vi "Read from memory.vi"(8 "input valid":bool=TRUE, 10 "Address":u32, 11 "Memory item":refnum<k21>="PID Output I") -> (0 "output valid":bool=TRUE, 2 "Address out":u32, 3 "Value out":fxp<+/-,32,14>)   [LabVIEW 2018]
uses:
  <vilib>/rvi/DataTransferAndStorage/Container/Common/niFpgaContainerExecOnDevCompGetState.vi
  <vilib>/rvi/Emulation/niFpgaEmulationIsFPGAContextNoSignature.vi
  <vilib>/rvi/DataTransferAndStorage/Container/Common/niFpgaContainerGetUniqueNameForEmu.vi
  <vilib>/rvi/Emulation/niFpgaProcessEmulError.vi
  <vilib>/rvi/Emulation/niFpgaSctlEmulationGetInTimedLoop.vi
  <vilib>/rvi/errors/nirviReportUnexpectedCaseInternalError (U32).vi
  <vilib>/rvi/Memory/Memory_Emulation/niFpgaMemoryEmulationCacheClearOnFirstRun.vi
  <vilib>/rvi/Memory/Memory_Emulation/nirvimemoryEmulationManagerCache_MakeExclusive.vi
  <vilib>/rvi/Memory/Memory_Emulation/niFpgaMemoryEmulationValidateCache.vi
  <vilib>/rvi/Memory/Memory_Emulation/nirvimemoryEmulationManagerCache_InsertValue.vi
  <vilib>/Utility/error.llb/Clear Errors.vi
  <vilib>/rvi/Memory/Memory_Emulation/nirvimemoryEmulationManagerCache_ReleaseExclusive.vi
  <vilib>/rvi/Memory/Memory_Emulation/nirvimemoryEmulationManagerCache_GetValue.vi
  <vilib>/rvi/Memory/Memory_Emulation/nirvimemoryEmulationManagerCache_SetValue.vi
  <vilib>/rvi/Emulation/niFpgaSctlEmulationResourceMgr.vi
  <vilib>/rvi/DataTransferAndStorage/Container/XNode/niFpgaContainer.xnode
  <vilib>/rvi/Memory/Memory_Emulation/niFpgaMemoryEmulationRefIn.vi
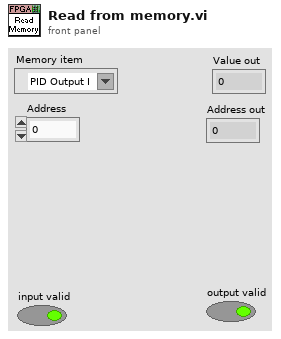
[diagram p1: front panel]
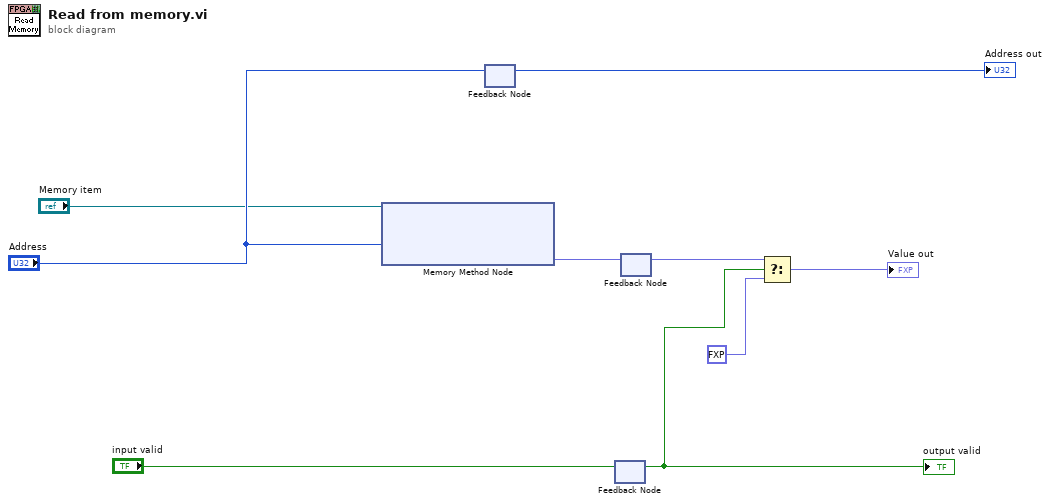
[diagram p0: block diagram]
diagram:
  n1 = xnode ("Memory Method Node")("Address"="Address", "Memory In"="Memory item") -> ("Data"=w9:fxp<+/-,32,14>)  [unwired: 1 out]
  n2 = feedback #1() -> (→"Address out":u32)  [unwired: 1 in]
  n3 = feedback-in #1("Address") -> ()
  n4 = feedback #2() -> (w1:bool)  [unwired: 1 in]
  "output valid" <- w1
  n5 = feedback-in #2("input valid") -> ()
  n6 = feedback-in #3(w9) -> ()
  n7 = feedback #3() -> (w7:fxp<+/-,32,14>)  [unwired: 1 in]
  n8 = Select(t=w7, s=w1, f=fxp<+/-,32,14> 0.0) -> (s? t:f=→"Value out":fxp<+/-,32,14>)
